vi "Database Interface Tests.vi"() -> ()   [LabVIEW 2020]
uses:
  source/Database OOP/Database Libraries/Database Interfaces/Column Information.ctl
  source/Database OOP/Database Libraries/Database Interfaces/Database data type.ctl
  source/Database OOP/Database Libraries/Database Interfaces/Primary Key Info.ctl
  source/Database OOP/Database Libraries/ADODB/ADODB Class/ADODB.lvclass
  source/Database OOP/Database Libraries/ADODB/UDL Connection Class/UDL Connection.lvclass
  C:/Users/User/Desktop/Raman Program/LV-Database-OOP/source/Database OOP/Database Libraries/Database Interfaces/Database Connection Class/Database Connection.lvclass
  source/Database OOP/Database Libraries/Database Interfaces.lvlib
panel:
  out "Primary Key Array":T1[](array[typedef])
  out "Provider Name":string
  out "Timestamp":string[](array[string])
  out "Column Information Array 2":T2[](array[typedef])
  out "Column Information Array":T2[](array[typedef])
  out "Foreign Key Array":T4(array[cluster])
  out "Column Name Array":string[](array[string])
  out "Table Names":string[](array[string])
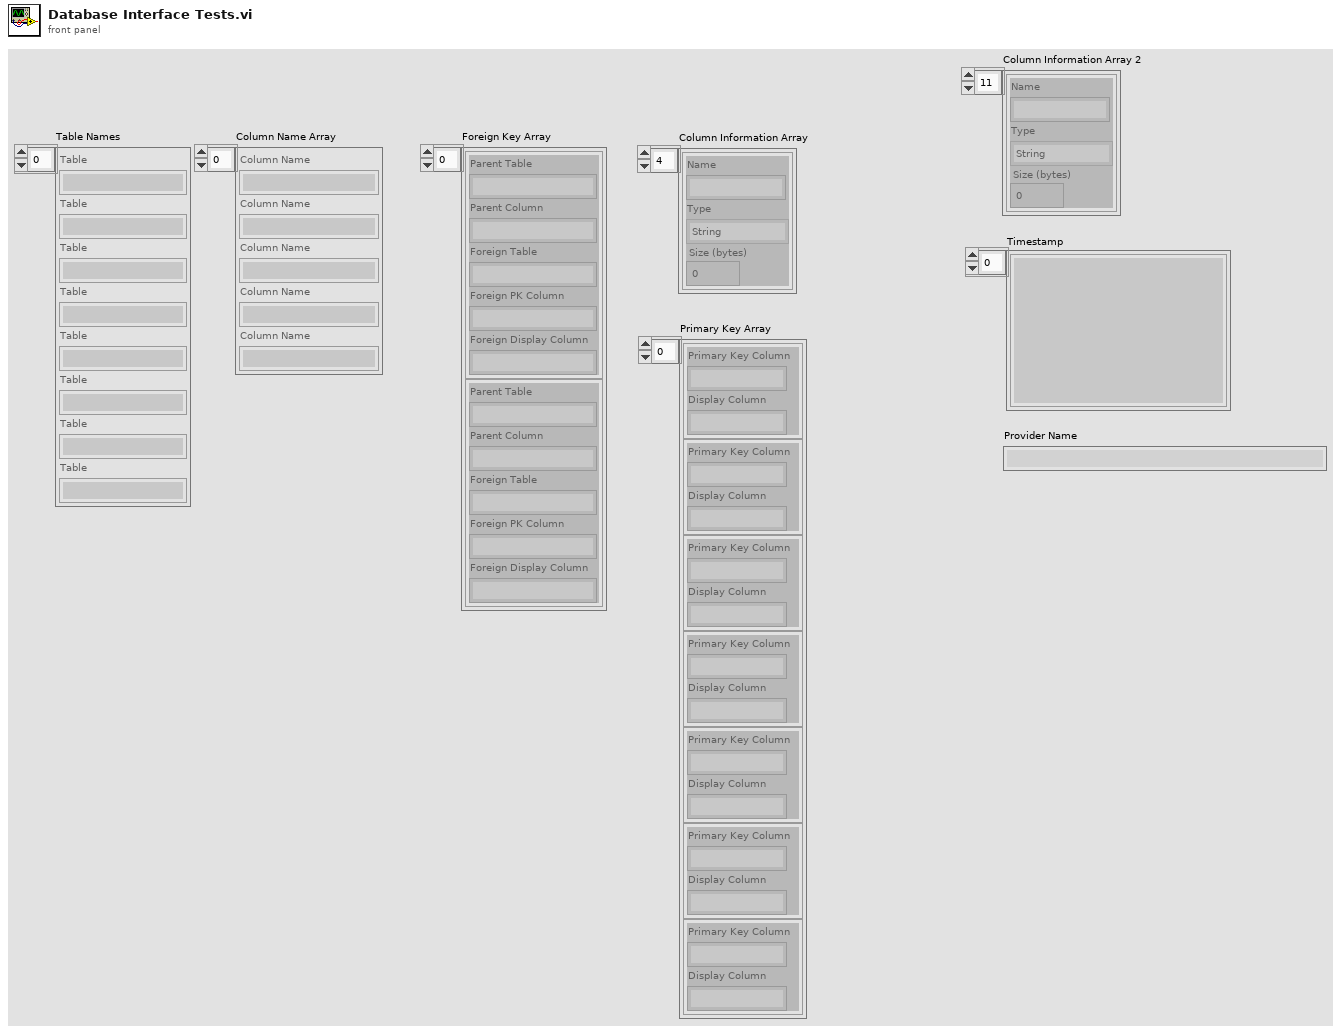
[diagram p1: front panel]
types:
  T1 = typedef "Database Interfaces.lvlib/Primary Key Info.ctl" = cluster{"Primary Key Column":string, "Display Column":string}
  T2 = typedef "Database Interfaces.lvlib/Column Information.ctl" = cluster{"Name":string, "Type":T3, "Size (bytes)":i32}
  T3 = typedef "Database Interfaces.lvlib/Database data type.ctl" = enum16{"Undefined", "String", "Long (I32)", "Single (SGL)", "Double (DBL)", "Date/Time", "Binary"}
  T4 = cluster{"Parent Table":string, "Parent Column":string, "Foreign Table":string, "Foreign PK Column":string, "Foreign Display Column":string}[]
  T5 = typedef "Database Interfaces.lvlib/foreign key properties.ctl" = cluster{"FK Table":string, "FK Column":string, "PK Table":string, "PK Column":string, "PK Display Column":string}
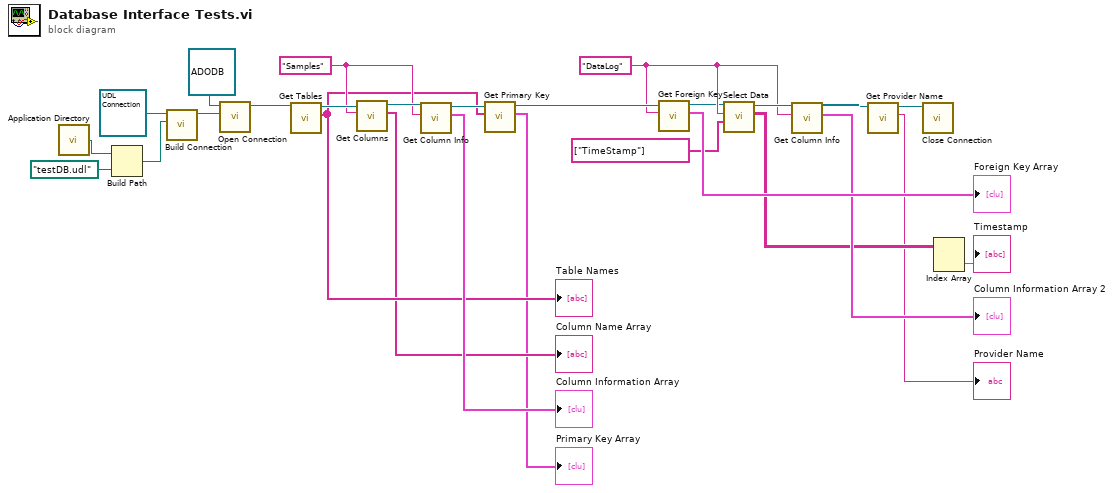
[diagram p0: block diagram]
diagram:
  w13 = "DataLog" ("Table Name")
  w24 = "Samples" ("Table Name")
  n1 = call <vilib>:"Application Directory.vi"() -> ("Application Directory"=w1:path)
  n2 = Build Path(base path=w1, name or relative path=path "testDB.udl") -> (appended path=w2:path)
  n3 = call "Build Connection.vi"("*.udl file path"=w2, "UDL Connection in"=refnum<class "UDL Connection.lvclass"> refnum ("ADODB.lvlib:UDL Connection.lvclass")) -> ("UDL Connection out"=w21:refnum<class "UDL Connection.lvclass">)  [unwired: 8 in, 1 out]
  n4 = call-dynamic "Open Connection.vi"("Connection"=w21, "ADODB in"=refnum<class "ADODB.lvclass"> refnum ("ODBC in")) -> ("ADODB out"=w27:refnum<class "ADODB.lvclass">)  [unwired: 8 in, 1 out]
  n5 = call-dynamic "Get Tables.vi"("ODBC in"=w27) -> ("Table Names"=w16:string[], "ODBC out"=w26:refnum<class "ADODB.lvclass">)  [unwired: 8 in, 1 out]
  "Table Names" <- w16
  n6 = call-dynamic "Get Columns.vi"("Table Name"=w24, "ADODB in"=w26) -> ("Column Name Array"=→"Column Name Array":string[], "ADODB out"=w25:refnum<class "ADODB.lvclass">)  [unwired: 7 in, 1 out]
  n7 = call-dynamic "Get Column Info.vi"("Table Name"=w24, "ODBC in"=w25) -> ("Column Information Array"=→"Column Information Array":T2[], "ODBC out"=w18:refnum<class "ADODB.lvclass">)  [unwired: 7 in, 1 out]
  n8 = call-dynamic "Get Primary Key.vi"("Table Name Array"=w16, "ADODB in"=w18) -> ("Primary Key Array"=→"Primary Key Array":T1[], "ADODB out"=w17:refnum<class "ADODB.lvclass">)  [unwired: 6 in, 2 out]
  n9 = call-dynamic "Get Foreign Key.vi"("Table Name"=w13, "ADODB in"=w17) -> ("FK Properties Array"=→"Foreign Key Array":T5[], "ADODB out"=w11:refnum<class "ADODB.lvclass">)  [unwired: 7 in, 1 out]
  n10 = call-dynamic "Select Data.vi"("Columns"=string[] ["TimeStamp"], "Table"=w13, "ADODB in"=w11) -> ("Data"=w9:string[][], "ADODB out"=w14:refnum<class "ADODB.lvclass">)  [unwired: 6 in, 1 out]
  n11 = call-dynamic "Get Column Info.vi"("Table Name"=w13, "ODBC in"=w14) -> ("Column Information Array"=→"Column Information Array 2":T2[], "ODBC out"=w7:refnum<class "ADODB.lvclass">)  [unwired: 7 in, 1 out]
  n12 = call-dynamic "Get Provider Name.vi"("ADODB in"=w7) -> ("Provider Name"=→"Provider Name":string, "ADODB out"=w6:refnum<class "ADODB.lvclass">)  [unwired: 8 in, 1 out]
  n13 = call-dynamic "Close Connection.vi"("ODBC in"=w6) -> ()  [unwired: 9 in, 2 out]
  n14 = Index Array(array=w9) -> (element=→"Timestamp":string[])  [unwired: 2 in]
